vi "Execute.vi"(8 "error in (no error)":errorcluster, 10 "Plugin Load Next in":refnum<class "Plugin Load Next.lvclass">, 11 "Plugin Handler Shifter Data Definition":T1) -> (0 "error out":errorcluster, 1 "Stop?":bool, 2 "Plugin Generic Command out":refnum<class "Plugin Handler Command.lvclass">, 3 "Plugin Handler Shifter Data Out":T1)   [LabVIEW 2011, in "Plugin Load Next.lvclass"]
uses:
  Plugin Load Next.lvclass
  Plugin Handler Command.lvclass
  Plugin Strict Type Definitions/Plugin Handler Shifter Data Definition.ctl
  Parent Plugin Definition/Plugin Template/Generic Plugin.lvclass
  Plugin Strict Type Definitions/Plugin Configuration Information.ctl
  User Interface/UI Command Manager/UI Command Manager.lvclass
  Plugin Display UI/Plugin Display UI.lvclass
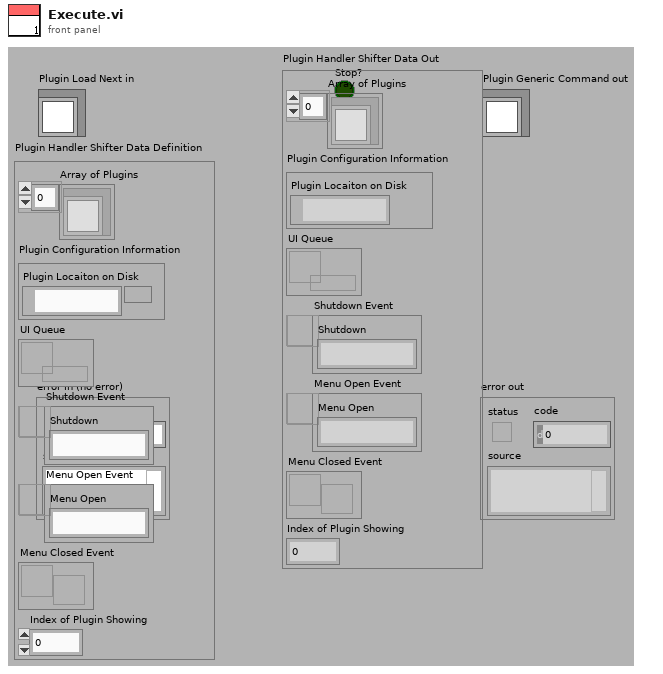
[diagram p1: front panel]
types:
  T1 = typedef "Plugin Handler Shifter Data Definition.ctl" = cluster{"Array of Plugins":refnum<class "Generic Plugin.lvclass">[], "Plugin Configuration Information":T2, "UI Queue":refnum<queue>, "Shutdown Event":refnum<user-event>, "Menu Open Event":refnum<user-event>, "Menu Closed Event":refnum<user-event>, "Index of Plugin Showing":i32}
  T2 = typedef "Plugin Configuration Information.ctl" = cluster{"Plugin Locaiton on Disk":path}
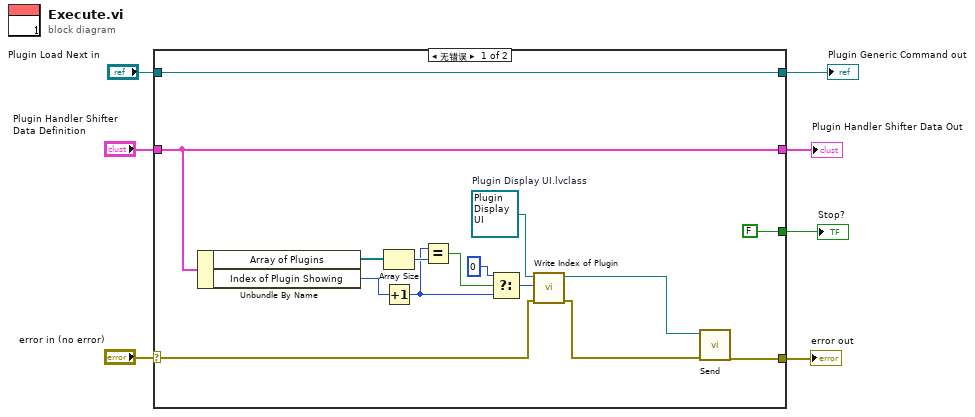
[diagram p0: block diagram]
diagram:
  n1 = case shown="无错误" "error in (no error)" {
    selector: "error in (no error)" -> [w11 w25]
    tunnel: "Plugin Handler Shifter Data Definition" -> [w8 w24]
    tunnel: [w16 w25] -> w6
    tunnel: [w8 w24] -> w2
    tunnel: "Plugin Load Next in" -> [w9 w23]
    tunnel: [w9 w23] -> w3
    tunnel: [FALSE ("Stop?") _] -> w1
    frame No Error {
      w14 = refnum<class "Plugin Display UI.lvclass"> refnum  # Plugin Display UI.lvclass
      n2 = Unbundle By Name(w8) -> ("Array of Plugins"=w21:refnum<class "Generic Plugin.lvclass">[], "Index of Plugin Showing"=w22:i32)
      n3 = Array Size(array=w21) -> (size(s)=w20:i32)
      n4 = Increment(x=w22) -> (x+1=w18:i32)
      n5 = Equal?(x=w18, y=w20) -> (x = y?=w19:bool)
      n6 = Select(t=0, s=w19, f=w18) -> (s? t:f=w15:i32)
      n7 = call "Write Index of Plugin.vi"("error in (no error)"=w11, "Index of Plugin"=w15, "Plugin Display UI in"=w14) -> ("error out"=w12:errorcluster, "Plugin Display UI out"=w13:refnum<class "Plugin Display UI.lvclass">)  [unwired: 7 in]
      n8 = call "Send.vi"("error in (no error)"=w12, "Plugin Generic Command in"=w13) -> ("error out"=w16:errorcluster)  [unwired: 8 in, 1 out]
    }
    frame Error {
    }
  }
  "error out" <- w6
  "Plugin Generic Command out" <- w3
  "Stop?" <- w1
  "Plugin Handler Shifter Data Out" <- w2
